vi "WebSocket Manerger(FGV).vi"(6 "WebSocket Manerger Method":T1=enum."Get Connections", 8 "error in":errorcluster, 11 "connection In":refnum<k5>) -> (0 "error out":errorcluster, 3 "connection Out":refnum<k5>[](array[refnum]))   [LabVIEW 2018]
uses:
  Data Def/WebSocket Manerger Method.ctl
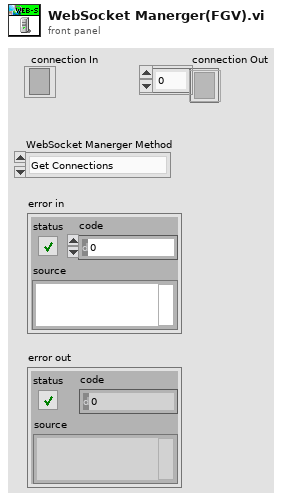
[diagram p1: front panel]
types:
  T1 = typedef "WebSocket Manerger Method.ctl" = enum16{"Initialize", "Add Connection", "Get Connections", "Close Connection", "Close All"}
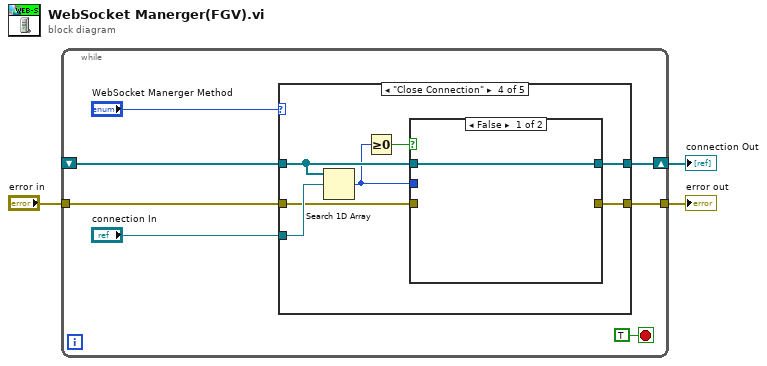
[diagram p0: block diagram]
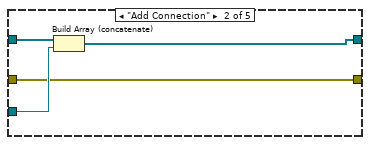
[diagram p3: hidden frame]
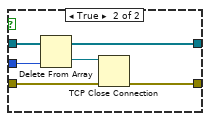
[diagram p5: hidden frame]
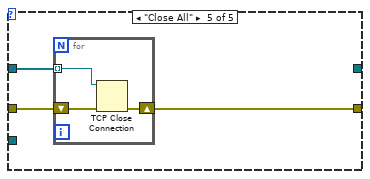
[diagram p6: hidden frame]
diagram:
  n1 = while {
    shift-right: [w7] -> w3
    shift-left: _ -> [w6]
    tunnel: "error in" -> [w5]
    tunnel: [w4] -> w1
    stop <- TRUE stop-if-true
    n2 = case shown="\"Close Connection\"" "WebSocket Manerger Method" {
      tunnel: "connection In" -> [_ w15 _ w24 _]
      tunnel: [_ w14 w17 w18 _] -> w7
      tunnel: w6 -> [_ w13 w17 w22 w32]
      tunnel: w5 -> [w11 w12 w16 w20 w34]
      tunnel: [w11 w12 w16 w19 w33] -> w4
      frame "Initialize", Default {
      }
      frame "Add Connection" {
        n3 = Build Array (concatenate)(w13, w15) -> (w14:refnum<k5>[])
      }
      frame "Get Connections" {
      }
      frame "Close Connection" {
        n4 = Search 1D Array(1D array=w22, element=w24) -> (index of element=w21:i32)  [unwired: 1 out]
        n5 = Greater Or Equal To 0?(x=w21) -> (x >= 0?=w23:bool)
        n6 = case shown="False" w23 {
          tunnel: w22 -> [w25 w31]
          tunnel: w21 -> [_ w30]
          tunnel: w20 -> [_ w29]
          tunnel: [_ w28] -> w19
          tunnel: [w25 w26] -> w18
          frame False {
          }
          frame True {
            n7 = Delete From Array(array=w31, index=w30) -> (deleted portion=w27:refnum<k5>, array with subset deleted=w26:refnum<k5>[])  [unwired: 1 in]
            n8 = TCP Close Connection(connection ID=w27, error in (no error)=w29) -> (error out=w28:errorcluster)  [unwired: 2 out]
          }
        }
      }
      frame "Close All" {
        n9 = for {
          tunnel: w32 -> [w37] mode=indexing
          shift-right: [w35] -> w33
          shift-left: w34 -> [w36]
          n10 = TCP Close Connection(connection ID=w37, error in (no error)=w36) -> (error out=w35:errorcluster)  [unwired: 2 out]
        }
      }
    }
  }
  "error out" <- w1
  "connection Out" <- w3
